vi "S2C_PCIe7841_Proc_Commands.vi"(7 "VI_Ref":refnum<vi>, 8 "Error In":errorcluster, 10 "Settings":T1, 11 "Q-Ref":refnum<queue>) -> (0 "Error Out":errorcluster, 2 "Stop?":bool, 3 "Response":variant)   [LabVIEW 2015]
uses:
  S2C_PCIe7841_Proc_Globals.vi
  _Shared/S2C_Shared_Proc_Globals.vi
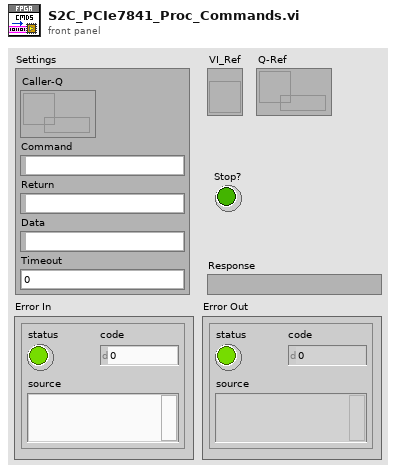
[diagram p1: front panel]
types:
  T1 = cluster{"Caller-Q":refnum<queue>, "Command":string, "Return":string, "Data":variant, "Timeout":dbl}
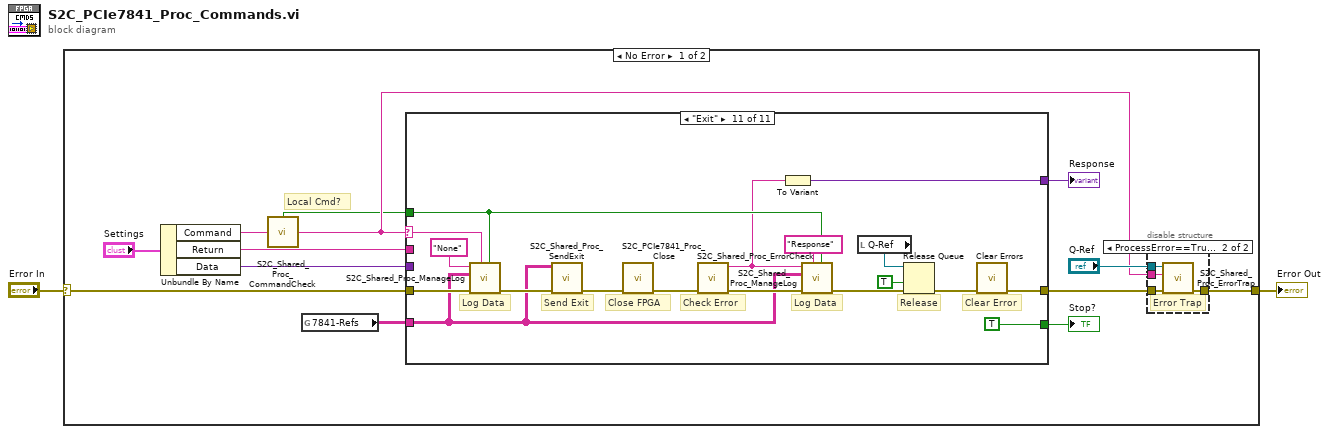
[diagram p0: block diagram]
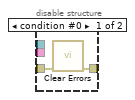
[diagram p2: hidden frame]
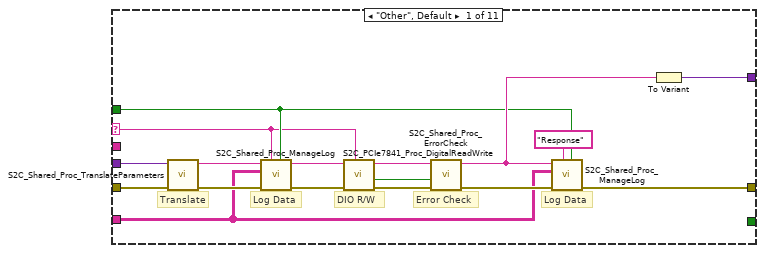
[diagram p3: hidden frame]
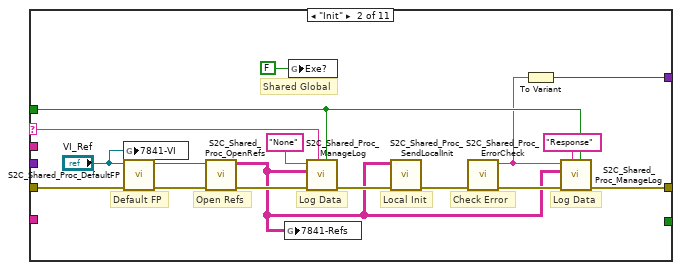
[diagram p4: hidden frame]
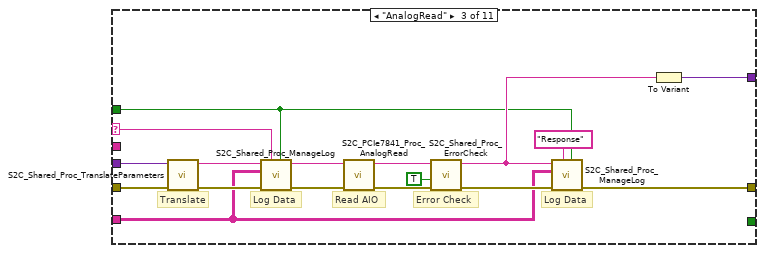
[diagram p5: hidden frame]
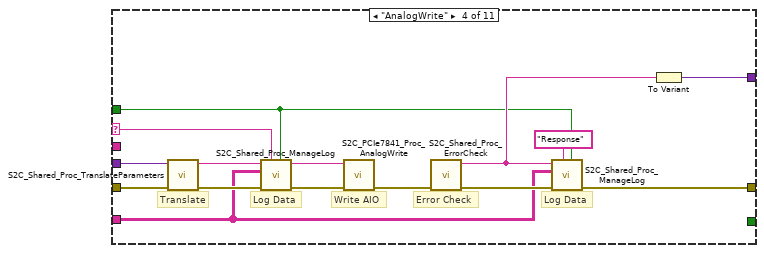
[diagram p6: hidden frame]
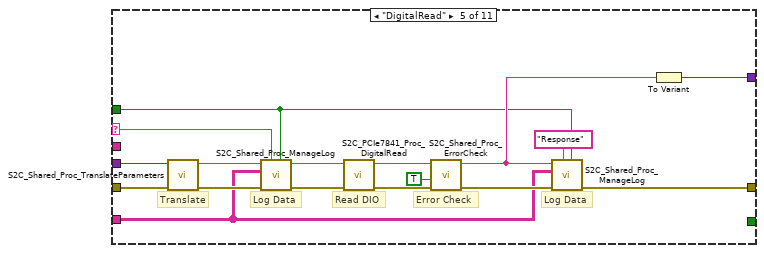
[diagram p7: hidden frame]
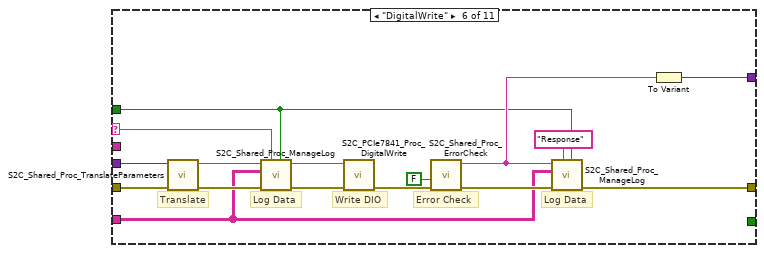
[diagram p8: hidden frame]
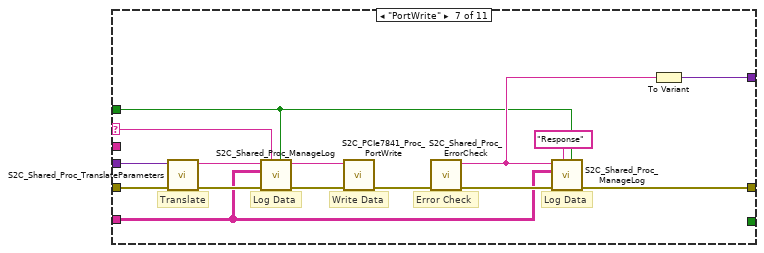
[diagram p9: hidden frame]
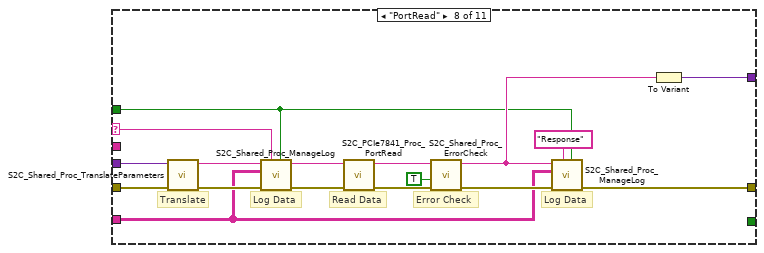
[diagram p10: hidden frame]
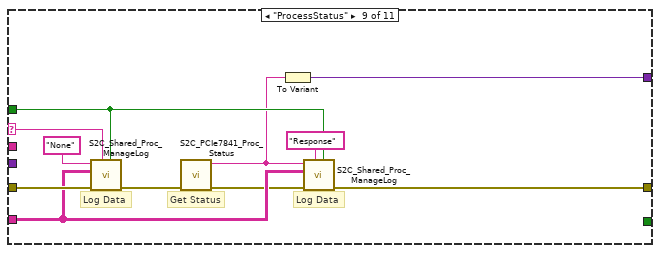
[diagram p11: hidden frame]
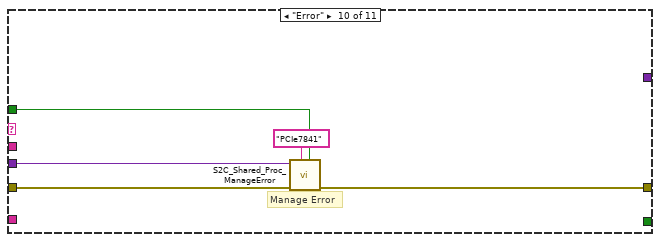
[diagram p12: hidden frame]
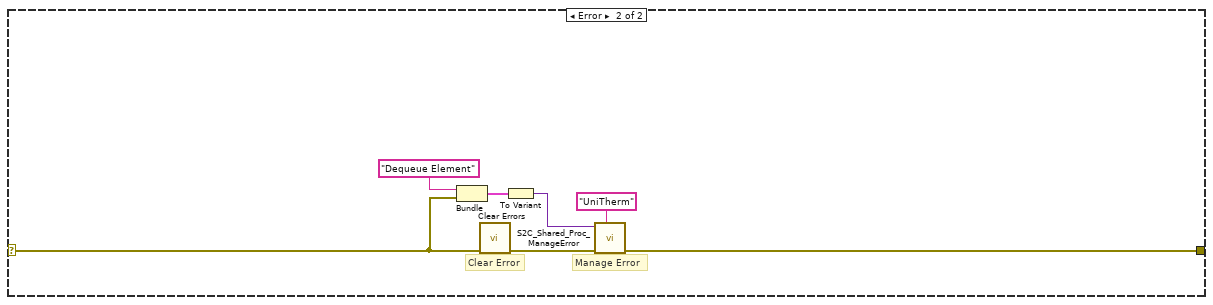
[diagram p13: hidden frame]
diagram:
  n1 = case shown="No Error" "Error In" {
    selector: "Error In" -> [w14 w190]
    tunnel: [w7 w192] -> w1
    frame No Error {
      # "Local Cmd?"
      n2 = Unbundle By Name("Settings") -> ("Command"=w6:string, "Return"=w10:string, "Data"=w15:variant)
      n3 = call "S2C_Shared_Proc_CommandCheck.vi"("Cmd In"=w6) -> ("Local?"=w4:bool, "Cmd Out"=w5:string)  [unwired: 13 in]
      n4 = global read "S2C_PCIe7841_Proc_Globals.vi" "7841-Refs"() -> (w3:string[][])
      n5 = case shown="\"Exit\"" w5 {
        selector: w5 -> [w24 w52 w59 w74 w91 w107 w122 w139 w162 _ w183]
        tunnel: w14 -> [w38 w45 w72 w87 w104 w120 w135 w152 w161 w167 w184]
        tunnel: w15 -> [w37 _ w71 w86 w103 w119 w134 w151 _ w164 _]
        tunnel: [w27 w55 w61 w76 w93 w109 w124 w141 w158 w166 w171] -> w8
        tunnel: [w28 w49 w62 w77 w94 w110 w125 w142 w159 _ w178] -> w12
        tunnel: [_ _ _ _ _ _ _ _ _ _ TRUE] -> w11
        tunnel: w10 -> [_ _ _ _ _ _ _ _ _ _ _]
        tunnel: w4 -> [w25 w53 w58 w73 w90 w106 w121 w138 w156 w165 w182]
        tunnel: w3 -> [w26 _ w60 w75 w92 w108 w123 w140 w157 _ w175]
        frame "Other", Default {
          # "DIO R/W"
          # "Error Check"
          # "Log Data"
          # "Log Data"
          # "Translate"
          n6 = call "S2C_Shared_Proc_TranslateParameters.vi"("Error In"=w38, "Data"=w37) -> ("Error Out"=w35:errorcluster, "JSON Cluster"=w36:string)  [unwired: 8 in]
          n7 = call "S2C_Shared_Proc_ManageLog.vi"("Local?"=w25, "Command"=w24, "Error In"=w35, "Refs"=w26, "Data In"=w36) -> ("Error Out"=w33:errorcluster, "Data Out"=w34:string)  [unwired: 5 in]
          n8 = call "S2C_PCIe7841_Proc_DigitalReadWrite.vi"("Command"=w24, "Error In"=w33, "Data In"=w34) -> ("Error Out"=w30:errorcluster, "ExpReply?"=w22:bool, "Data Out"=w23:string)  [unwired: 6 in]
          n9 = call "S2C_Shared_Proc_ErrorCheck.vi"("Error In"=w30, "ExpReply?"=w22, "Reply Text"=w23) -> ("Error Out"=w31:errorcluster, "Status"=w29:string)  [unwired: 7 in]
          n10 = call "S2C_Shared_Proc_ManageLog.vi"("Local?"=w25, "Command"="Response", "Error In"=w31, "Refs"=w26, "Data In"=w29) -> ("Error Out"=w27:errorcluster)  [unwired: 5 in, 1 out]
          n11 = To Variant(anything=w29) -> (Variant=w28:variant)
        }
        frame "Init" {
          # "Local Init"
          # "Default FP"
          # "Shared Global"
          # "Check Error"
          # "Log Data"
          # "Open Refs"
          # "Log Data"
          n12 = global write "S2C_PCIe7841_Proc_Globals.vi" "7841-VI"("VI_Ref") -> ()
          n13 = call "S2C_Shared_Proc_DefaultFP.vi"("Error In"=w45, "VI_Ref In"="VI_Ref") -> ("Error Out"=w43:errorcluster, "VI_Ref Out"=w44:refnum<vi>)  [unwired: 8 in]
          n14 = call "S2C_Shared_Proc_OpenRefs.vi"("Error In"=w43, "VI_Ref"=w44) -> ("Error Out"=w46:errorcluster, "Refs"=w39:string[][])  [unwired: 8 in]
          n15 = global write "S2C_PCIe7841_Proc_Globals.vi" "7841-Refs"(w39) -> ()
          n16 = global write "S2C_Shared_Proc_Globals.vi" "Exe?"(FALSE ("Exe?")) -> ()
          n17 = call "S2C_Shared_Proc_ManageLog.vi"("Local?"=w53, "Command"=w52, "Error In"=w46, "Refs"=w39, "Data In"="None") -> ("Error Out"=w41:errorcluster)  [unwired: 5 in, 1 out]
          n18 = call "S2C_Shared_Proc_SendLocalInit.vi"("Error In"=w41, "Refs"=w39) -> ("Error Out"=w40:errorcluster)  [unwired: 9 in]
          n19 = call "S2C_Shared_Proc_ErrorCheck.vi"("Error In"=w40) -> ("Error Out"=w50:errorcluster, "Status"=w48:string)  [unwired: 9 in]
          n20 = To Variant(anything=w48) -> (Variant=w49:variant)
          n21 = call "S2C_Shared_Proc_ManageLog.vi"("Local?"=w53, "Command"="Response", "Error In"=w50, "Refs"=w39, "Data In"=w48) -> ("Error Out"=w55:errorcluster)  [unwired: 5 in, 1 out]
        }
        frame "AnalogRead" {
          # "Read AIO"
          # "Error Check"
          # "Log Data"
          # "Log Data"
          # "Translate"
          n22 = call "S2C_Shared_Proc_TranslateParameters.vi"("Error In"=w72, "Data"=w71) -> ("Error Out"=w69:errorcluster, "JSON Cluster"=w70:string)  [unwired: 8 in]
          n23 = call "S2C_Shared_Proc_ManageLog.vi"("Local?"=w58, "Command"=w59, "Error In"=w69, "Refs"=w60, "Data In"=w70) -> ("Error Out"=w67:errorcluster, "Data Out"=w68:string)  [unwired: 5 in]
          n24 = call "S2C_PCIe7841_Proc_AnalogRead.vi"("Error In"=w67, "Data"=w68) -> ("Error Out"=w64:errorcluster, "Result"=w57:string)  [unwired: 8 in]
          n25 = call "S2C_Shared_Proc_ErrorCheck.vi"("Error In"=w64, "ExpReply?"=TRUE, "Reply Text"=w57) -> ("Error Out"=w65:errorcluster, "Status"=w63:string)  [unwired: 7 in]
          n26 = call "S2C_Shared_Proc_ManageLog.vi"("Local?"=w58, "Command"="Response", "Error In"=w65, "Refs"=w60, "Data In"=w63) -> ("Error Out"=w61:errorcluster)  [unwired: 5 in, 1 out]
          n27 = To Variant(anything=w63) -> (Variant=w62:variant)
        }
        frame "AnalogWrite" {
          # "Write AIO"
          # "Error Check"
          # "Log Data"
          # "Log Data"
          # "Translate"
          n28 = call "S2C_Shared_Proc_TranslateParameters.vi"("Error In"=w87, "Data"=w86) -> ("Error Out"=w84:errorcluster, "JSON Cluster"=w85:string)  [unwired: 8 in]
          n29 = call "S2C_Shared_Proc_ManageLog.vi"("Local?"=w73, "Command"=w74, "Error In"=w84, "Refs"=w75, "Data In"=w85) -> ("Error Out"=w82:errorcluster, "Data Out"=w83:string)  [unwired: 5 in]
          n30 = call "S2C_PCIe7841_Proc_AnalogWrite.vi"("Error In"=w82, "Data"=w83) -> ("Error Out"=w79:errorcluster)  [unwired: 9 in]
          n31 = call "S2C_Shared_Proc_ErrorCheck.vi"("Error In"=w79) -> ("Error Out"=w80:errorcluster, "Status"=w78:string)  [unwired: 9 in]
          n32 = call "S2C_Shared_Proc_ManageLog.vi"("Local?"=w73, "Command"="Response", "Error In"=w80, "Refs"=w75, "Data In"=w78) -> ("Error Out"=w76:errorcluster)  [unwired: 5 in, 1 out]
          n33 = To Variant(anything=w78) -> (Variant=w77:variant)
        }
        frame "DigitalRead" {
          # "Read DIO"
          # "Error Check"
          # "Log Data"
          # "Log Data"
          # "Translate"
          n34 = call "S2C_Shared_Proc_TranslateParameters.vi"("Error In"=w104, "Data"=w103) -> ("Error Out"=w101:errorcluster, "JSON Cluster"=w102:string)  [unwired: 8 in]
          n35 = call "S2C_Shared_Proc_ManageLog.vi"("Local?"=w90, "Command"=w91, "Error In"=w101, "Refs"=w92, "Data In"=w102) -> ("Error Out"=w99:errorcluster, "Data Out"=w100:string)  [unwired: 5 in]
          n36 = call "S2C_PCIe7841_Proc_DigitalRead.vi"("Error In"=w99, "Data"=w100) -> ("Error Out"=w96:errorcluster, "Response"=w89:string)  [unwired: 8 in]
          n37 = call "S2C_Shared_Proc_ErrorCheck.vi"("Error In"=w96, "ExpReply?"=TRUE, "Reply Text"=w89) -> ("Error Out"=w97:errorcluster, "Status"=w95:string)  [unwired: 7 in]
          n38 = call "S2C_Shared_Proc_ManageLog.vi"("Local?"=w90, "Command"="Response", "Error In"=w97, "Refs"=w92, "Data In"=w95) -> ("Error Out"=w93:errorcluster)  [unwired: 5 in, 1 out]
          n39 = To Variant(anything=w95) -> (Variant=w94:variant)
        }
        frame "DigitalWrite" {
          # "Write DIO"
          # "Error Check"
          # "Log Data"
          # "Log Data"
          # "Translate"
          n40 = call "S2C_Shared_Proc_TranslateParameters.vi"("Error In"=w120, "Data"=w119) -> ("Error Out"=w117:errorcluster, "JSON Cluster"=w118:string)  [unwired: 8 in]
          n41 = call "S2C_Shared_Proc_ManageLog.vi"("Local?"=w106, "Command"=w107, "Error In"=w117, "Refs"=w108, "Data In"=w118) -> ("Error Out"=w115:errorcluster, "Data Out"=w116:string)  [unwired: 5 in]
          n42 = call "S2C_PCIe7841_Proc_DigitalWrite.vi"("Error In"=w115, "Data"=w116) -> ("Error Out"=w112:errorcluster)  [unwired: 9 in]
          n43 = call "S2C_Shared_Proc_ErrorCheck.vi"("Error In"=w112, "ExpReply?"=FALSE) -> ("Error Out"=w113:errorcluster, "Status"=w111:string)  [unwired: 8 in]
          n44 = call "S2C_Shared_Proc_ManageLog.vi"("Local?"=w106, "Command"="Response", "Error In"=w113, "Refs"=w108, "Data In"=w111) -> ("Error Out"=w109:errorcluster)  [unwired: 5 in, 1 out]
          n45 = To Variant(anything=w111) -> (Variant=w110:variant)
        }
        frame "PortWrite" {
          # "Write Data"
          # "Error Check"
          # "Log Data"
          # "Log Data"
          # "Translate"
          n46 = call "S2C_Shared_Proc_TranslateParameters.vi"("Error In"=w135, "Data"=w134) -> ("Error Out"=w132:errorcluster, "JSON Cluster"=w133:string)  [unwired: 8 in]
          n47 = call "S2C_Shared_Proc_ManageLog.vi"("Local?"=w121, "Command"=w122, "Error In"=w132, "Refs"=w123, "Data In"=w133) -> ("Error Out"=w130:errorcluster, "Data Out"=w131:string)  [unwired: 5 in]
          n48 = call "S2C_PCIe7841_Proc_PortWrite.vi"("Error In"=w130, "Data"=w131) -> ("Error Out"=w127:errorcluster)  [unwired: 9 in]
          n49 = call "S2C_Shared_Proc_ErrorCheck.vi"("Error In"=w127) -> ("Error Out"=w128:errorcluster, "Status"=w126:string)  [unwired: 9 in]
          n50 = call "S2C_Shared_Proc_ManageLog.vi"("Local?"=w121, "Command"="Response", "Error In"=w128, "Refs"=w123, "Data In"=w126) -> ("Error Out"=w124:errorcluster)  [unwired: 5 in, 1 out]
          n51 = To Variant(anything=w126) -> (Variant=w125:variant)
        }
        frame "PortRead" {
          # "Read Data"
          # "Error Check"
          # "Log Data"
          # "Log Data"
          # "Translate"
          n52 = call "S2C_Shared_Proc_TranslateParameters.vi"("Error In"=w152, "Data"=w151) -> ("Error Out"=w149:errorcluster, "JSON Cluster"=w150:string)  [unwired: 8 in]
          n53 = call "S2C_Shared_Proc_ManageLog.vi"("Local?"=w138, "Command"=w139, "Error In"=w149, "Refs"=w140, "Data In"=w150) -> ("Error Out"=w147:errorcluster, "Data Out"=w148:string)  [unwired: 5 in]
          n54 = call "S2C_PCIe7841_Proc_PortRead.vi"("Error In"=w147, "Data"=w148) -> ("Error Out"=w144:errorcluster, "Port"=w137:string)  [unwired: 8 in]
          n55 = call "S2C_Shared_Proc_ErrorCheck.vi"("Error In"=w144, "ExpReply?"=TRUE, "Reply Text"=w137) -> ("Error Out"=w145:errorcluster, "Status"=w143:string)  [unwired: 7 in]
          n56 = call "S2C_Shared_Proc_ManageLog.vi"("Local?"=w138, "Command"="Response", "Error In"=w145, "Refs"=w140, "Data In"=w143) -> ("Error Out"=w141:errorcluster)  [unwired: 5 in, 1 out]
          n57 = To Variant(anything=w143) -> (Variant=w142:variant)
        }
        frame "ProcessStatus" {
          # "Get Status"
          # "Log Data"
          # "Log Data"
          n58 = call "S2C_Shared_Proc_ManageLog.vi"("Local?"=w156, "Command"=w162, "Error In"=w161, "Refs"=w157, "Data In"="None") -> ("Error Out"=w155:errorcluster)  [unwired: 5 in, 1 out]
          n59 = call "S2C_PCIe7841_Proc_Status.vi"("Error In"=w155) -> ("Error Out"=w154:errorcluster, "Response"=w153:string)  [unwired: 9 in]
          n60 = To Variant(anything=w153) -> (Variant=w159:variant)
          n61 = call "S2C_Shared_Proc_ManageLog.vi"("Local?"=w156, "Command"="Response", "Error In"=w154, "Refs"=w157, "Data In"=w153) -> ("Error Out"=w158:errorcluster)  [unwired: 5 in, 1 out]
        }
        frame "Error" {
          # "Manage Error"
          n62 = call "S2C_Shared_Proc_ManageError.vi"("Local?"=w165, "Process"="PCIe7841", "Error In"=w167, "Data"=w164) -> ("Error Out"=w166:errorcluster)  [unwired: 7 in]
        }
        frame "Exit" {
          # "Close FPGA"
          # "Clear Error"
          # "Release"
          # "Check Error"
          # "Send Exit"
          # "Log Data"
          # "Log Data"
          n63 = call "S2C_Shared_Proc_ManageLog.vi"("Local?"=w182, "Command"=w183, "Error In"=w184, "Refs"=w175, "Data In"="None") -> ("Error Out"=w176:errorcluster)  [unwired: 5 in, 1 out]
          n64 = call "S2C_Shared_Proc_SendExit.vi"("Error In"=w176, "Refs"=w175) -> ("Error Out"=w170:errorcluster)  [unwired: 9 in]
          n65 = call "S2C_PCIe7841_Proc_Close.vi"("Error In"=w170) -> ("Error Out"=w169:errorcluster)  [unwired: 10 in]
          n66 = call "S2C_Shared_Proc_ErrorCheck.vi"("Error In"=w169) -> ("Error Out"=w180:errorcluster, "Status"=w177:string)  [unwired: 9 in]
          n67 = To Variant(anything=w177) -> (Variant=w178:variant)
          n68 = call "S2C_Shared_Proc_ManageLog.vi"("Local?"=w182, "Command"="Response", "Error In"=w180, "Refs"=w175, "Data In"=w177) -> ("Error Out"=w179:errorcluster)  [unwired: 5 in, 1 out]
          n69 = local read "Q-Ref"() -> (w173:refnum<queue>)
          n70 = Release Queue(queue=w173, force destroy? (F)=TRUE, error in (no error)=w179) -> (error out=w174:errorcluster)  [unwired: 2 out]
          n71 = call <vilib>:"Clear Errors.vi"("error in (no error)"=w174) -> ("error out"=w171:errorcluster)  [unwired: 5 in, 1 out]
        }
      }
      "Response" <- w12
      "Stop?" <- w11
      n72 = disable-structure shown="ProcessError==True" {
        disable-tunnel: w8 -> [w17 w21]
        disable-tunnel: [w16 w20] -> w7
        disable-tunnel: w5 -> [_ w19]
        disable-tunnel: "Q-Ref" -> [_ w18]
        frame condition #0 {
          n73 = call <vilib>:"Clear Errors.vi"("error in (no error)"=w17) -> ("error out"=w16:errorcluster)  [unwired: 5 in, 1 out]
        }
        frame condition #1 (active) {
          # "Error Trap"
          n74 = call "S2C_Shared_Proc_ErrorTrap.vi"("Error In"=w21, "Command"=w19, "Q-Ref"=w18) -> ("Error Out"=w20:errorcluster)  [unwired: 8 in]
        }
      }
    }
    frame Error {
      # "Clear Error"
      # "Manage Error"
      n75 = Bundle("Dequeue Element", "error IO"=w190) -> (w191:cluster{string, "error IO":errorcluster})  [unwired: 1 in]
      n76 = call <vilib>:"Clear Errors.vi"("error in (no error)"=w190) -> ("error out"=w187:errorcluster)  [unwired: 5 in, 1 out]
      n77 = To Variant(anything=w191) -> (Variant=w188:variant)
      n78 = call "S2C_Shared_Proc_ManageError.vi"("Process"="UniTherm", "Error In"=w187, "Data"=w188) -> ("Error Out"=w192:errorcluster)  [unwired: 8 in]
    }
  }
  "Error Out" <- w1
